vi "Raise Stop Event.vi"(8 "error in (no error)":errorcluster, 9 "Raiser Id":string, 10 "Raiser Name":string, 11 "Send Stop":bool=TRUE) -> (0 "error out":errorcluster)   [LabVIEW 2023, in "HAF.lvlib"]
doc: "Helper member to send a Stop Event if the passed Boolean is True. It is always sent as high priority."
uses:
  HAF.lvlib
  Event Data.ctl
  <vilib>/event_ctls.llb/usereventprio.ctl
  Stop Event.ctl
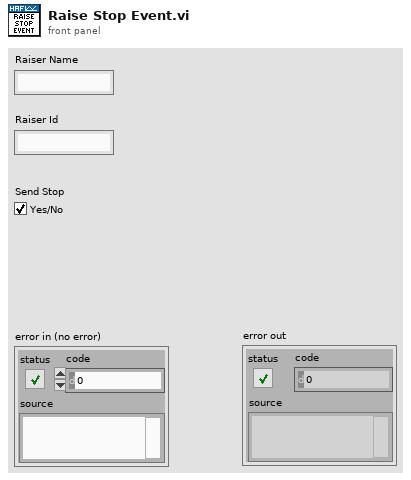
[diagram p1: front panel]
types:
  T1 = typedef "usereventprio.ctl" = enum32{"high priority", "normal priority"}
  T2 = typedef "HAF.lvlib/Event Data.ctl" = cluster{"Raiser Name":string, "Raiser Id":string}
  T3 = typedef "HAF.lvlib/Stop Event.ctl" = refnum<user-event>
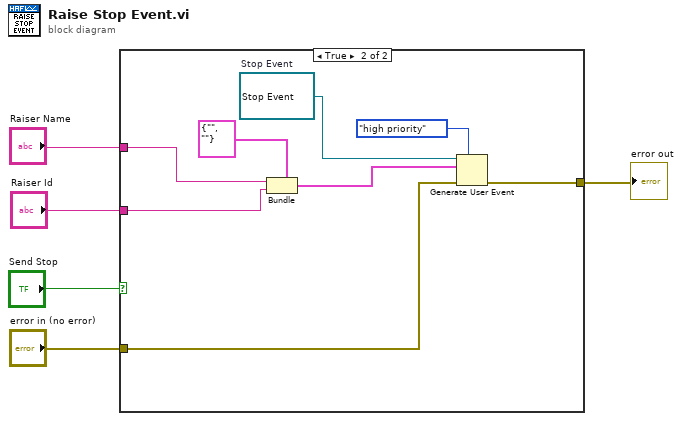
[diagram p0: block diagram]
diagram:
  n1 = case shown="True" "Send Stop" {
    tunnel: "error in (no error)" -> [w6 w10]
    tunnel: "Raiser Name" -> [_ w13]
    tunnel: "Raiser Id" -> [_ w12]
    tunnel: [w6 w9] -> w1
    frame False {
    }
    frame True {
      w7 = T3 refnum  # Stop Event
      n2 = Bundle(cluster=T2 {"Raiser Name"="", "Raiser Id"=""} ("Event Data Structure"), "Raiser Name"=w13, "Raiser Id"=w12) -> (w11:T2)
      n3 = Generate User Event(priority (normal)=usereventprio."high priority", user event=w7, event data cluster=w11, error in=w10) -> (error out=w9:errorcluster)  [unwired: 1 out]
    }
  }
  "error out" <- w1
